vi "Read_flag-state.vi"(8 "error in (no error)":errorcluster, 11 "flag in":refnum<class "flag.lvclass">) -> (0 "error out":errorcluster, 2 "flag state":bool, 3 "flag out":refnum<class "flag.lvclass">)   [LabVIEW 2018, in "flag.lvclass"]
uses:
  flag.lvclass
  flag.lvclass/flag.ctl
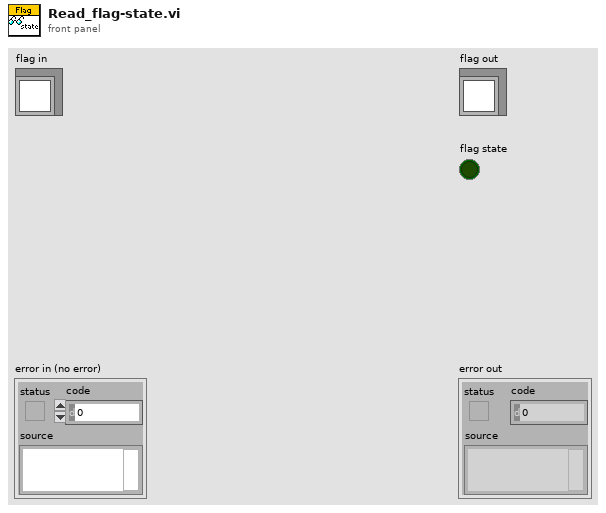
[diagram p1: front panel]
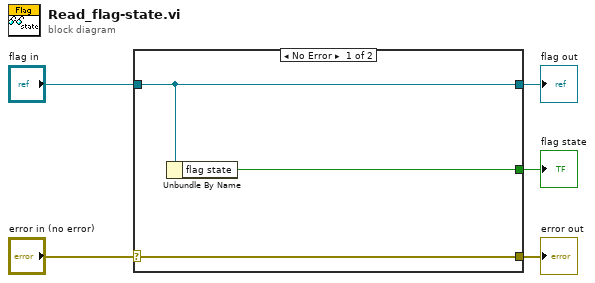
[diagram p0: block diagram]
diagram:
  n1 = case shown="No Error" "error in (no error)" {
    selector: "error in (no error)" -> [w8 w9]
    tunnel: [w8 w9] -> w4
    tunnel: [w7 w10] -> w2
    tunnel: "flag in" -> [w7 w10]
    tunnel: [w6 _] -> w1
    frame No Error {
      n2 = Unbundle By Name(w7) -> ("flag state"=w6:bool)
    }
    frame Error {
    }
  }
  "error out" <- w4
  "flag out" <- w2
  "flag state" <- w1
